vi "KlingerV2 SetStatusOptions.vi"(4 "error in":errorcluster, 6 "StatusOpt":T1={"AXIS MOVING"=TRUE, "W & X TRAVEL LIMIT"=TRUE, "Y & Z TRAVEL LIMIT"=TRUE, "INPUT BITS VALUE"=TRUE, "W  POSITION"=TRUE, "X  POSITION"=TRUE, "Y  POSITION"=TRUE, "Z  POSITION"=TRUE} caption="Status Report Options", 7 "VISA Rsrc":refnum<visa-resource-name>="SR530") -> (0 "error out":errorcluster)   [LabVIEW 2010]
doc: "Ce VI permet de régler les options de rapport de statut du contrôleur.Celle-ci détermines les informations qui seront envoyer lors d'une lecture ou à la suite de la commande \"?\""
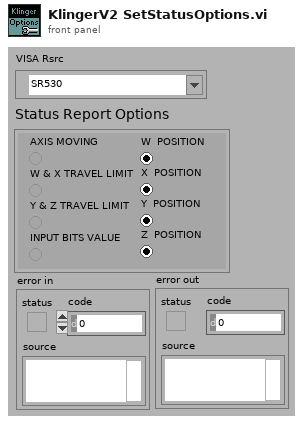
[diagram p1: front panel]
types:
  T1 = cluster{"AXIS MOVING":bool, "W & X TRAVEL LIMIT":bool, "Y & Z TRAVEL LIMIT":bool, "INPUT BITS VALUE":bool, "W  POSITION":bool, "X  POSITION":bool, "Y  POSITION":bool, "Z  POSITION":bool}
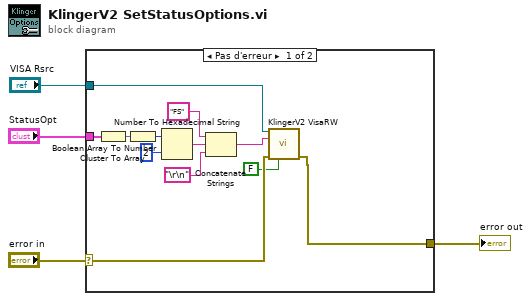
[diagram p0: block diagram]
diagram:
  n1 = case shown="Pas d'erreur" "error in" {
    tunnel: [w9 w17] -> w4
    tunnel: "StatusOpt" -> [w14 _]
    selector: "error in" -> [w8 w17]
    tunnel: "VISA Rsrc" -> [w6 _]
    frame No Error {
      n2 = Cluster To Array(cluster=w14) -> (array=w13:bool[])
      n3 = Boolean Array To Number(Boolean array=w13) -> (number=w12:u32)
      n4 = Number To Hexadecimal String(1:i16 2 ("width (-)"), 2:w12) -> (0:w11:string)
      n5 = Concatenate Strings("FS", w11, "\r\n") -> (w7:string)
      n6 = call <userlib>:"KlingerV2 VisaRW.vi"("VISA Rsrc"=w6, "ChaineCom"=w7, "error in (no error)"=w8, "Lecture?(T)"=FALSE) -> ("error out"=w9:errorcluster)  [unwired: 7 in, 4 out]
    }
    frame Error {
    }
  }
  "error out" <- w4
